vi "Modbus Master simulator.vi"   [LabVIEW 2020, in "Modbus.lvlib"]
uses:
  Modbus/Modbus.lvlib
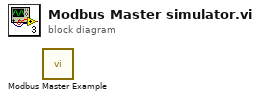
[diagram p0: block diagram]
diagram:
  n1 = call "Modbus Master Example.vi"() -> ()  [unwired: 12 in]
